vi "_CSMObj-Update CSMList.vi"(8 "Error In":errorcluster caption="error in (no error)", 11 "CSMObj In":T1) -> (0 "error out":errorcluster, 3 "CSMObj Out":T1)   [LabVIEW 2017, in "Communicable State Machine.lvlib"]
uses:
  Communicable State Machine.lvlib
  _CSMObj.ctl
  _CSMObj-Info.ctl
  Typedef/_CSM_MODE.ctl
  _CSMObj-Refs.ctl
  _CSMObj-Data.ctl
  Typedef/_CSM_MSG_TYPE.ctl
  Priority Queue/Priority Queue.ctl
  Typedef/_Cross CSM State Data.ctl
  Typedef/_Cross CSM State Response.ctl
  Typedef/_CSM_Response Source Message.ctl
  Priority Queue/def-Data(LowPRI-Q).ctl
  _CSMObj-ModeData.ctl
  Typedef/_CSM Status Change Event Data.ctl
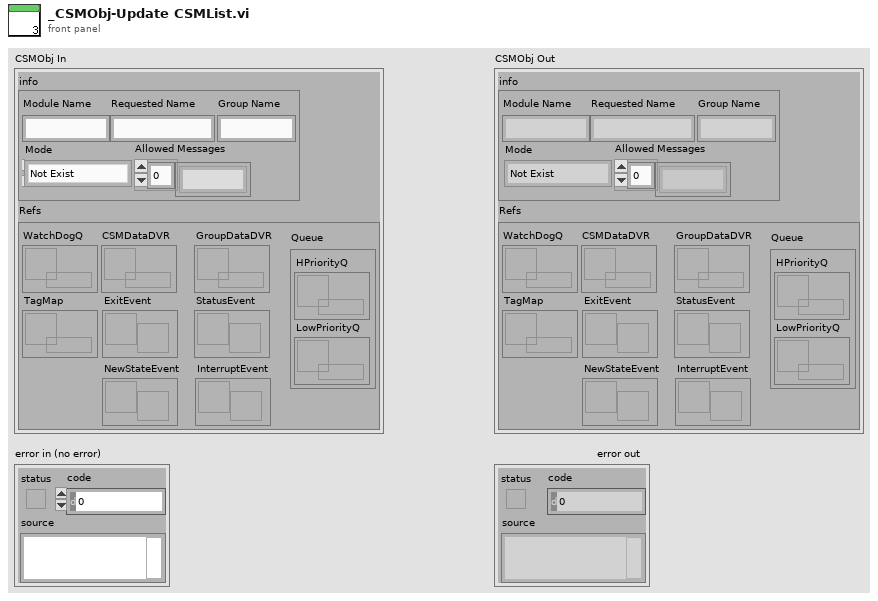
[diagram p1: front panel]
types:
  T1 = typedef "Communicable State Machine.lvlib/_CSMObj.ctl" = cluster{"info":T2, "Refs":T4}
  T2 = typedef "Communicable State Machine.lvlib/_CSMObj-Info.ctl" = cluster{"Module Name":string, "Requested Name":string, "Group Name":string, "Mode":T3, "Allowed Messages":string[]}
  T3 = typedef "Communicable State Machine.lvlib/_CSM_MODE.ctl" = enum16{"Not Exist", "Stand Alone", "CSM", "Worker", "Worker Agent", "Chain Node", "Chain"}
  T4 = typedef "Communicable State Machine.lvlib/_CSMObj-Refs.ctl" = cluster{"WatchDogQ":refnum<queue>, "CSMDataDVR":refnum<data-value>, "Queue":T5, "GroupDataDVR":refnum<data-value>, "TagMap":refnum<data-value>, "ExitEvent":refnum<user-event>, "NewStateEvent":refnum<user-event>, "StatusEvent":refnum<user-event>, "InterruptEvent":refnum<user-event>}
  T5 = typedef "Communicable State Machine.lvlib/Priority Queue.ctl" = cluster{"HPriorityQ":refnum<queue>, "LowPriorityQ":refnum<queue>}
  T6 = typedef "Communicable State Machine.lvlib/_CSMObj-ModeData.ctl" = cluster{"CSMDataDVR":refnum<data-value>[], "PriorityQueues":T5[], "Messages of Chain Nodes":cluster{"Module Name":string, "Allowed Messages":string[]}[], "Chain Message Mapping Map":variant, "SharedRegistryRules":string[]}
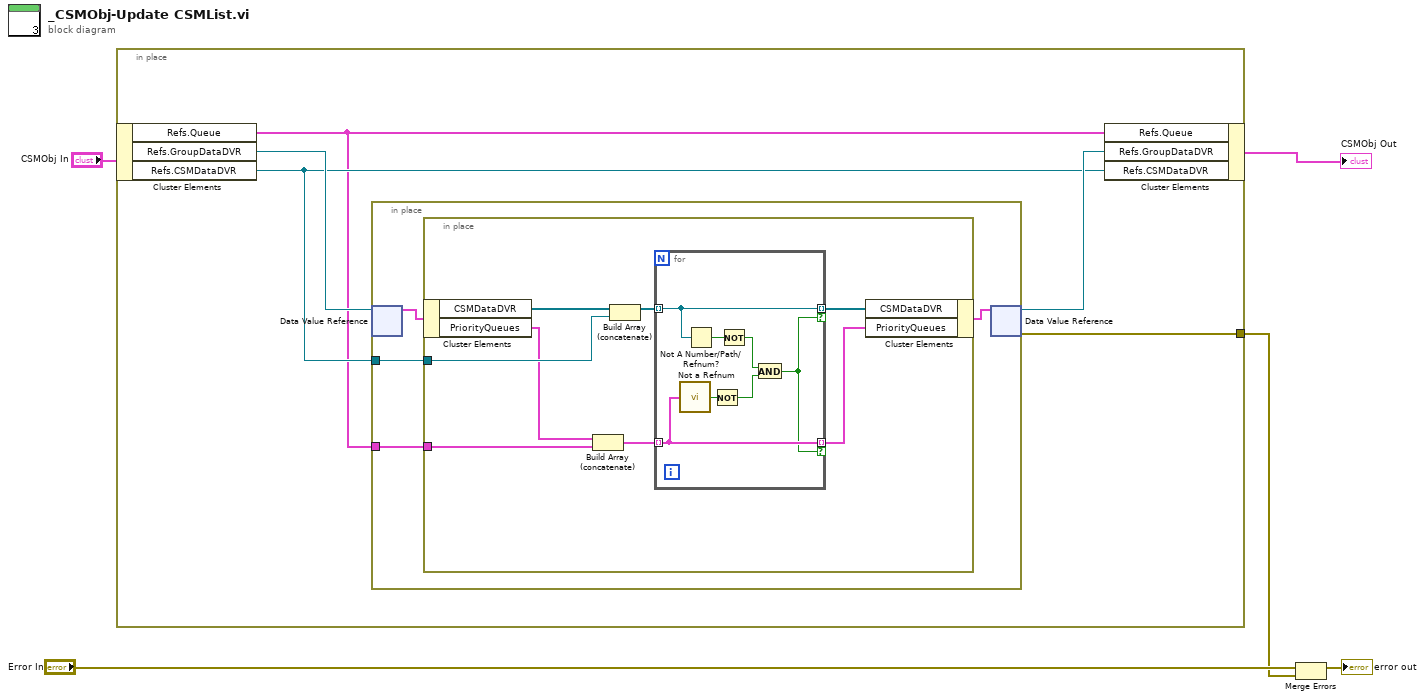
[diagram p0: block diagram]
diagram:
  n1 = in-place "In Place Element Structure" {
    in-place-border: [w7] -> w1
    n2 = in-place-cluster #1("CSMObj In") -> ("Refs.Queue"=w6:T5, "Refs.GroupDataDVR"=w9:refnum<data-value>, "Refs.CSMDataDVR"=w8:refnum<data-value>)
    n3 = in-place {
      in-place-border: w8 -> [w12]
      in-place-border: w6 -> [w11]
      n4 = in-place-dvr #2(w9) -> (w14:T6)  [unwired: 1 out]
      n5 = in-place {
        in-place-border: w12 -> [w21]
        in-place-border: w11 -> [w17]
        n6 = in-place-cluster #3(w14) -> ("CSMDataDVR"=w22:refnum<data-value>[], "PriorityQueues"=w18:T5[])
        n7 = Build Array (concatenate)(w18, w17) -> (w16:T5[])
        n8 = Build Array (concatenate)(w22, w21) -> (w19:refnum<data-value>[])
        n9 = for {
          tunnel: [w29] -> w20 mode=indexing if=w23
          tunnel: w19 -> [w29] mode=indexing
          tunnel: w16 -> [w26] mode=indexing
          tunnel: [w26] -> w15 mode=indexing if=w23
          n10 = call "Not a Refnum.vi"("Priority Queue.lvclass"=w26) -> ("NaN/Path/Refnum?"=w27:bool)  [unwired: 4 in]
          n11 = Not A Number/Path/Refnum?(number/path/refnum=w29) -> (NaN/Path/Refnum?=w28:bool)
          n12 = Not(x=w27) -> (.not. x?=w24:bool)
          n13 = Not(x=w28) -> (.not. x?=w25:bool)
          n14 = And(x=w25, y=w24) -> (x .and. y?=w23:bool)
        }
        n15 = in-place-cluster #3("CSMDataDVR"=w20, "PriorityQueues"=w15) -> (w13:T6)
      }
      n16 = in-place-dvr #2(w13) -> (w10:refnum<data-value>, w7:errorcluster)
    }
    n17 = in-place-cluster #1("Refs.Queue"=w6, "Refs.GroupDataDVR"=w10, "Refs.CSMDataDVR"=w8) -> (→"CSMObj Out":T1)
  }
  n18 = Merge Errors("Error In", w1) -> (→"error out":errorcluster)
